vi "Init Bank DAQ.vi"(4 "Trigger source":tag="/Dev1/PFI0", 5 "pretrigger samples per channel":u32=20000, 6 "Sample rate":dbl=2000000.0 format="%.2p", 7 "samples per channel":i32=220000, 8 "Error In":errorcluster, 9 "input terminal configuration":i32(ring)=10106 items=["default"=-1, "RSE"=10083, "NRSE"=10078, "Differential"=10106, "Pseudodifferential"=12529], 10 "Range":dbl=10.0, 11 "physical channels":tag="Dev1/ai0:7") -> (0 "Error Out":errorcluster, 3 "task out":refnum<k21>)   [LabVIEW 2015, in "NHMFL User Bank.lvlib"]
uses:
  NHMFL User Bank.lvlib
  <vilib>/DAQmx/create/channels.llb/DAQmx Create Channel (AI-Voltage-Basic).vi
  <vilib>/DAQmx/configure/timing.llb/DAQmx Timing (Sample Clock).vi
  <vilib>/DAQmx/configure/trigger.llb/DAQmx Reference Trigger (Digital Edge).vi
  <resource>/objmgr/daqmx.rc
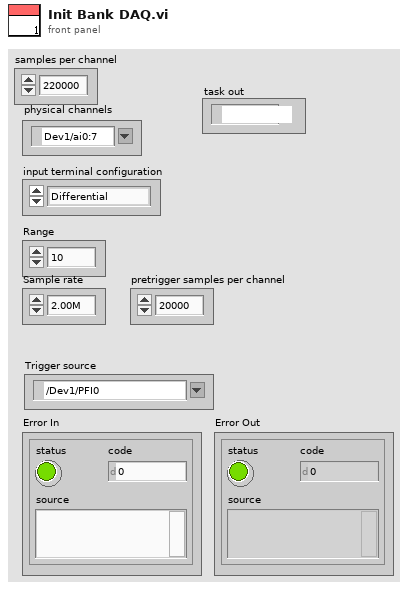
[diagram p1: front panel]
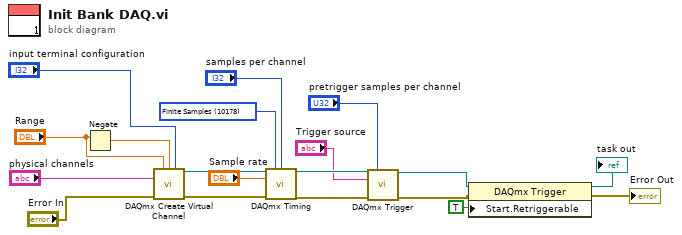
[diagram p0: block diagram]
diagram:
  w11 = 10178 items=["Finite Samples"=10178, "Continuous Samples"=10123, "Hardware Timed Single Point"=12522] ("sample mode")
  n1 = Negate(x="Range") -> (-x=w17:dbl)
  n2 = call-poly <vilib>:"DAQmx Create Virtual Channel.vi"("maximum value"="Range", "minimum value"=w17, "input terminal configuration"="input terminal configuration", "physical channels"="physical channels", "error in"="Error In") -> ("task out"=w15:refnum<k21>, "error out"=w14:errorcluster)  [unwired: 4 in, 5 out]
  n3 = call-poly <vilib>:"DAQmx Timing.vi"("task/channels in"=w15, "sample mode"=w11, "samples per channel"="samples per channel", "rate"="Sample rate", "error in"=w14) -> ("task out"=w10:refnum<k21>, "error out"=w9:errorcluster)  [unwired: 9 in]
  n4 = call-poly <vilib>:"DAQmx Trigger.vi"("task/channels in"=w10, "source"="Trigger source", "error in"=w9, "pretrigger samples per channel"="pretrigger samples per channel") -> ("task out"=w4:refnum<k21>, "error out"=w5:errorcluster)  [unwired: 1 in, 9 out]
  n5 = property class="DAQmx Trigger"(reference=w4, error in=w5, "Start.Retriggerable"=TRUE) -> (reference out=→"task out":refnum<k21>, error out=→"Error Out":errorcluster)
